vi "Convert Trace to RAW Frame.vi"() -> ()   [LabVIEW 2025, in "CAN-LIN Raw Bus Capture UI.lvlib"]
uses:
  <vilib>/xnet/xnet.llb/XNET Frame CAN.ctl
  <vilib>/xnet/xnet.llb/XNET Frame Type CAN.ctl
  CAN-LIN Raw Bus Capture UI.lvlib
panel:
  in  "payload":u8[](array[numeric])
  out "raw frames":u8[](array[numeric]) format="%02x"
  in  "captured data in":string[][](array[string])
  in  "bus type in":string
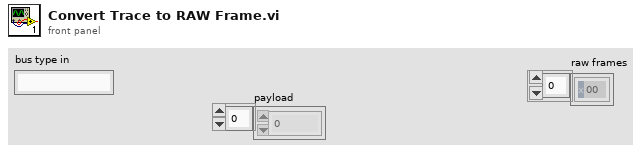
[diagram p1: front panel]
types:
  T1 = typedef "XNET Frame CAN.ctl" = cluster{"timestamp":timestamp, "payload":u8[], "identifier":u32, "type":T2, "extended?":bool, "echo?":bool}
  T2 = typedef "XNET Frame Type CAN.ctl" = u8
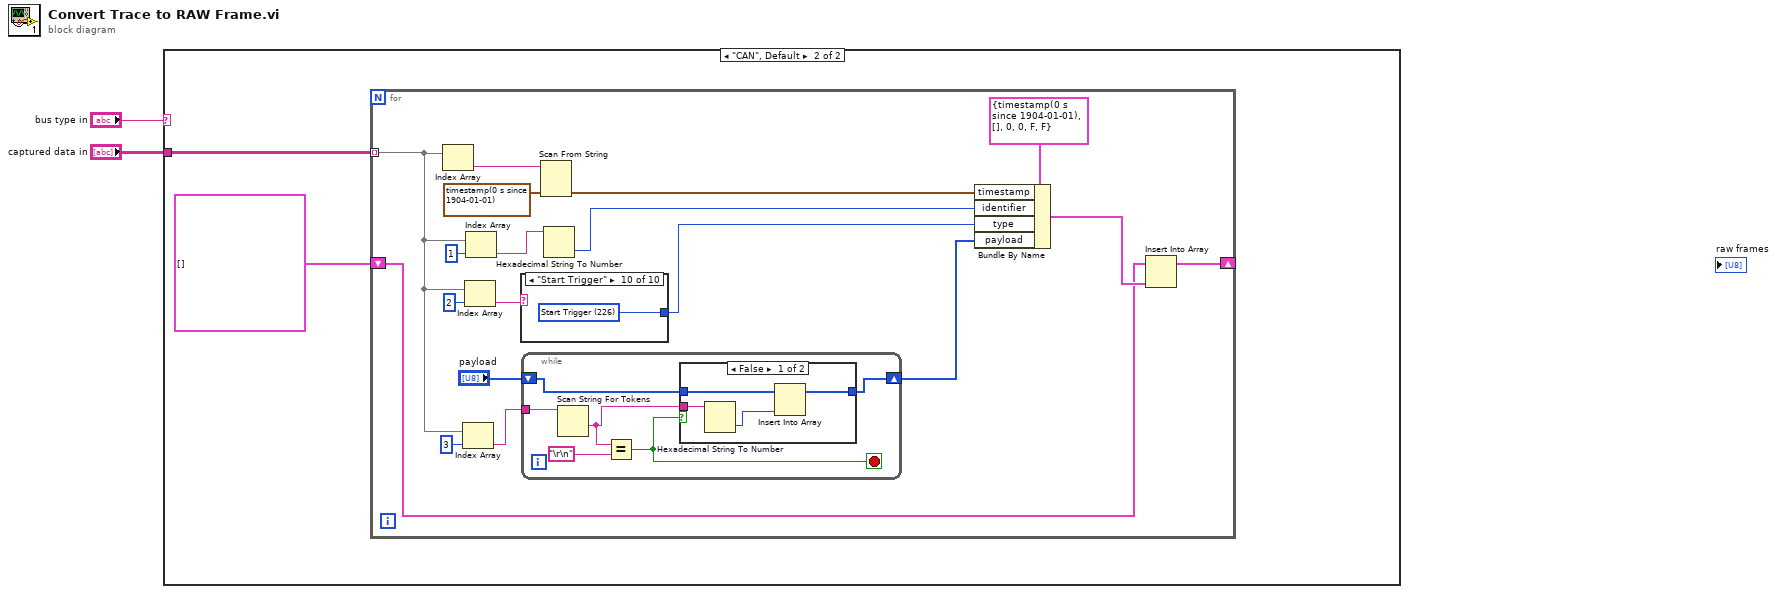
[diagram p0: block diagram]
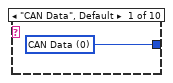
[diagram p4: hidden frame]
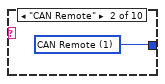
[diagram p5: hidden frame]
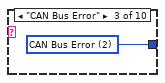
[diagram p6: hidden frame]
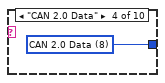
[diagram p7: hidden frame]
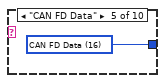
[diagram p8: hidden frame]
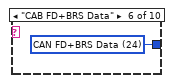
[diagram p9: hidden frame]
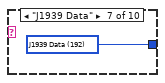
[diagram p10: hidden frame]
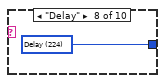
[diagram p11: hidden frame]
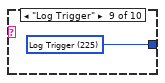
[diagram p12: hidden frame]
diagram:
  n1 = case shown="\"CAN\", Default" "bus type in" {
    tunnel: "captured data in" -> [_ w4]
    frame "False" {
    }
    frame "CAN", Default {
      n2 = for {
        tunnel: w4 -> [w9] mode=indexing
        shift-right: [w19] -> _
        shift-left: T1[] [] ("CAN frames") -> [w20]
        n3 = Index Array(array=w9) -> (element=w17:string)  [unwired: 1 in]
        n4 = Index Array(array=w9, index=3) -> (element=w7:string)
        n5 = Index Array(array=w9, index=2) -> (element=w11:string)
        n6 = Index Array(array=w9, index=1) -> (element=w14:string)
        n7 = case shown="\"Start Trigger\"" w11 {
          tunnel: [w34 w35 w36 w37 w38 w39 w40 w41 w42 w43] -> w10
          frame "CAN Data", Default {
            w34 = T2 0 items=["CAN Data"=0, "CAN Remote"=1, "CAN Bus Error"=2, "CAN 2.0 Data"=8, "CAN FD Data"=16, "CAN FD+BRS Data"=24, "J1939 Data"=192, "Delay"=224, "Log Trigger"=225, "Start Trigger"=226] ("type")
          }
          frame "CAN Remote" {
            w35 = T2 1 items=["CAN Data"=0, "CAN Remote"=1, "CAN Bus Error"=2, "CAN 2.0 Data"=8, "CAN FD Data"=16, "CAN FD+BRS Data"=24, "J1939 Data"=192, "Delay"=224, "Log Trigger"=225, "Start Trigger"=226] ("type")
          }
          frame "CAN Bus Error" {
            w36 = T2 2 items=["CAN Data"=0, "CAN Remote"=1, "CAN Bus Error"=2, "CAN 2.0 Data"=8, "CAN FD Data"=16, "CAN FD+BRS Data"=24, "J1939 Data"=192, "Delay"=224, "Log Trigger"=225, "Start Trigger"=226] ("type")
          }
          frame "CAN 2.0 Data" {
            w37 = T2 8 items=["CAN Data"=0, "CAN Remote"=1, "CAN Bus Error"=2, "CAN 2.0 Data"=8, "CAN FD Data"=16, "CAN FD+BRS Data"=24, "J1939 Data"=192, "Delay"=224, "Log Trigger"=225, "Start Trigger"=226] ("type")
          }
          frame "CAN FD Data" {
            w38 = T2 16 items=["CAN Data"=0, "CAN Remote"=1, "CAN Bus Error"=2, "CAN 2.0 Data"=8, "CAN FD Data"=16, "CAN FD+BRS Data"=24, "J1939 Data"=192, "Delay"=224, "Log Trigger"=225, "Start Trigger"=226] ("type")
          }
          frame "CAB FD+BRS Data" {
            w39 = T2 24 items=["CAN Data"=0, "CAN Remote"=1, "CAN Bus Error"=2, "CAN 2.0 Data"=8, "CAN FD Data"=16, "CAN FD+BRS Data"=24, "J1939 Data"=192, "Delay"=224, "Log Trigger"=225, "Start Trigger"=226] ("type")
          }
          frame "J1939 Data" {
            w40 = T2 192 items=["CAN Data"=0, "CAN Remote"=1, "CAN Bus Error"=2, "CAN 2.0 Data"=8, "CAN FD Data"=16, "CAN FD+BRS Data"=24, "J1939 Data"=192, "Delay"=224, "Log Trigger"=225, "Start Trigger"=226] ("type")
          }
          frame "Delay" {
            w41 = T2 224 items=["CAN Data"=0, "CAN Remote"=1, "CAN Bus Error"=2, "CAN 2.0 Data"=8, "CAN FD Data"=16, "CAN FD+BRS Data"=24, "J1939 Data"=192, "Delay"=224, "Log Trigger"=225, "Start Trigger"=226] ("type")
          }
          frame "Log Trigger" {
            w42 = T2 225 items=["CAN Data"=0, "CAN Remote"=1, "CAN Bus Error"=2, "CAN 2.0 Data"=8, "CAN FD Data"=16, "CAN FD+BRS Data"=24, "J1939 Data"=192, "Delay"=224, "Log Trigger"=225, "Start Trigger"=226] ("type")
          }
          frame "Start Trigger" {
            w43 = T2 226 items=["CAN Data"=0, "CAN Remote"=1, "CAN Bus Error"=2, "CAN 2.0 Data"=8, "CAN FD Data"=16, "CAN FD+BRS Data"=24, "J1939 Data"=192, "Delay"=224, "Log Trigger"=225, "Start Trigger"=226] ("type")
          }
        }
        n8 = while {
          tunnel: w7 -> [w28]
          shift-right: [w24] -> w5
          shift-left: "payload" -> [w25]
          stop <- w26 stop-if-true
          n9 = Scan String For Tokens(9:w28) -> (1:w23:string)  [unwired: 5 in, 3 out]
          n10 = Equal?(x=w23, y="\r\n") -> (x = y?=w26:bool)
          n11 = case shown="False" w26 {
            tunnel: w25 -> [w31 w33]
            tunnel: [w29 w33] -> w24
            tunnel: w23 -> [w32 _]
            frame False {
              n12 = Hexadecimal String To Number(string=w32) -> (number=w30:u32)  [unwired: 2 in, 1 out]
              n13 = Insert Into Array(array=w31, new element=w30) -> (w29:u8[])  [unwired: 1 in]
            }
            frame True {
            }
          }
        }
        n14 = Scan From String(input string=w17, default 1=timestamp(0 s since 1904-01-01) ("timestamp")) -> (output 1=w16:timestamp)  [unwired: 3 in, 3 out]
        n15 = Hexadecimal String To Number(string=w14) -> (number=w13:u32)  [unwired: 2 in, 1 out]
        n16 = Bundle By Name(cluster=T1 {"timestamp"=timestamp(0 s since 1904-01-01), "payload"=[], "identifier"=0, "type"=0, "extended?"=FALSE, "echo?"=FALSE} ("CAN frame"), "timestamp"=w16, "identifier"=w13, "type"=w10, "payload"=w5) -> (w21:T1)
        n17 = Insert Into Array(array=w20, new element=w21) -> (w19:T1[])  [unwired: 1 in]
      }
    }
  }
